vi "RT Driver VI.vi"(7 "Operation":T1, 11 "Device Reference in":T2 format="%.0x") -> (0 "Error Code":i32)   [LabVIEW 2020, in "AIM ARINC 429 Engine.lvlib" / "Custom Device.lvlib"]
uses:
  Custom Device.lvlib
  <vilib>/NI/NIVS Inline Async API/_VS Inline Async API/VS Inline Async API/VS Inline Async API.lvclass
  <vilib>/NI VeriStand/Custom Device API/Custom Device API.lvlib
  <vilib>/NI VeriStand/Custom Device Tools/Custom Device Utility Library/Custom Device Utility Library.lvlib
  <vilib>/NI VeriStand/Custom Device API/Data Reference.ctl
  <vilib>/NI VeriStand/Custom Device API/Block Data Reference.ctl
  Inline Execution Unit Runtime Information.ctl
  RTStateVariables.ctl
  Asynchronous Execution Unit Runtime Information.ctl
  Interfaces/Execution Unit/Execution Unit.lvclass
  Scripting/AIM/Constants.vi
  Scripting/AIM/AIM ARINC 429 Scripting.lvlib
  Inline Execution Unit Compiled Information.ctl
  Asynchronous Execution Unit Compiled Information.ctl
  Compiled.Settings.ctl
  <vilib>/NI VeriStand/Custom Device API/Get Item Property (Variant).vi
  Interfaces/Shared Resources/Shared Resources.lvclass
  <vilib>/NI VeriStand/Custom Device API/Custom Device Item Ref.ctl
  <vilib>/NI VeriStand/Custom Device API/Hardware Interface Driver VI Operation.ctl
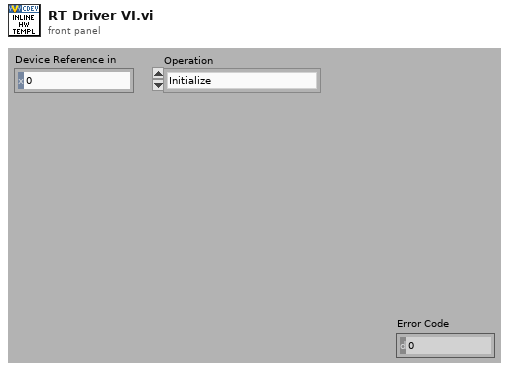
[diagram p1: front panel]
types:
  T1 = typedef "Custom Device API.lvlib/Hardware Interface Driver VI Operation.ctl" = enum16{"Initialize", "Start", "Read Data from HW", "Write Data to HW", "Close"}
  T2 = typedef "Custom Device API.lvlib/Custom Device Item Ref.ctl" = u64
  T3 = typedef "AIM ARINC 429 Engine.lvlib/Custom Device.lvlib/RTStateVariables.ctl" = cluster{"Async":refnum<class "VS Inline Async API.lvclass">, "Inline Execution Units":T4[], "Asynchronous Execution Units":T7[], "shared resources":refnum<class "Shared Resources.lvclass">}
  T4 = typedef "AIM ARINC 429 Engine.lvlib/Custom Device.lvlib/Inline Execution Unit Runtime Information.ctl" = cluster{"Execution Unit":refnum<class "Execution Unit.lvclass">, "Incoming Buffer":dbl[], "Outgoing Buffer":dbl[], "Incoming Data References":T5[], "Outgoing Data References":T6[]}
  T5 = typedef "Custom Device API.lvlib/Data Reference.ctl" = i32
  T6 = typedef "Custom Device API.lvlib/Block Data Reference.ctl" = cluster{"Data Reference":T5, "Offset":u64, "Length":u64}
  T7 = typedef "AIM ARINC 429 Engine.lvlib/Custom Device.lvlib/Asynchronous Execution Unit Runtime Information.ctl" = cluster{"Execution Unit":refnum<class "Execution Unit.lvclass">, "Incoming Channel Group Name":string, "Outgoing Channel Group Name":string, "ReadWrite Channel Group Name":string}
  T8 = typedef "AIM ARINC 429 Engine.lvlib/Custom Device.lvlib/Compiled.Settings.ctl" = cluster{"Name":string, "Inline Execution Unit Compiled Information":T9[], "Asynchronous Execution Unit Compiled Information":T10[], "flattened shared resources":string}
  T9 = typedef "AIM ARINC 429 Engine.lvlib/Custom Device.lvlib/Inline Execution Unit Compiled Information.ctl" = cluster{"Flattened Execution Unit":string, "Incoming Buffer":dbl[], "Outgoing Buffer":dbl[], "Incoming Data References":T5[], "Outgoing Data References":T6[]}
  T10 = typedef "AIM ARINC 429 Engine.lvlib/Custom Device.lvlib/Asynchronous Execution Unit Compiled Information.ctl" = cluster{"Flattened Execution Unit":string, "Incoming Channel Group Name":string, "Outgoing Channel Group Name":string, "ReadWrite Channel Group Name":string}
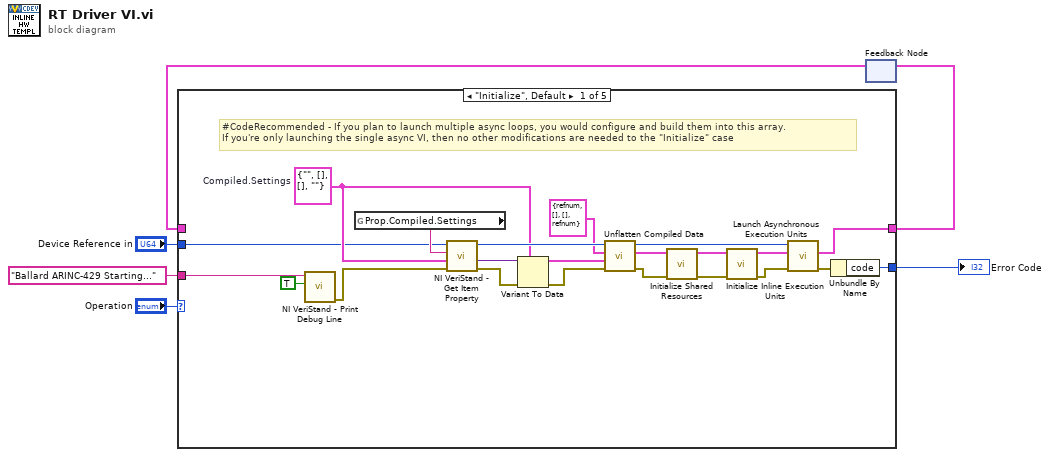
[diagram p0: block diagram]
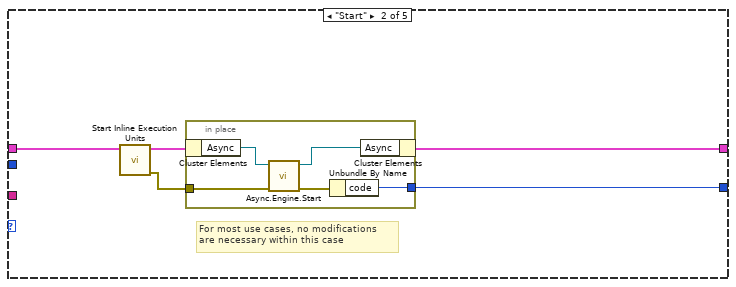
[diagram p2: hidden frame]
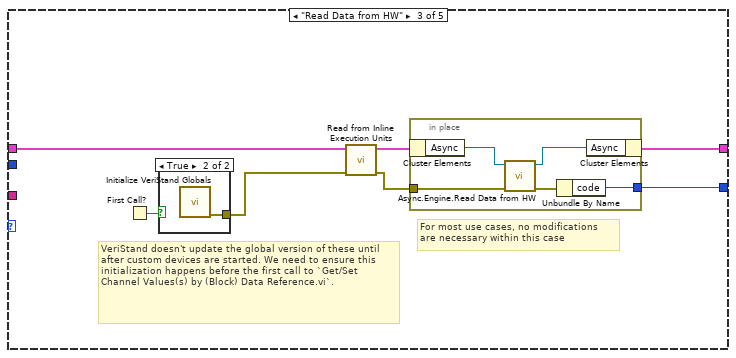
[diagram p3: hidden frame]
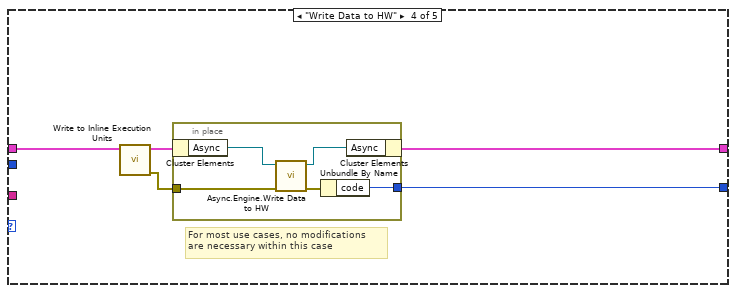
[diagram p5: hidden frame]
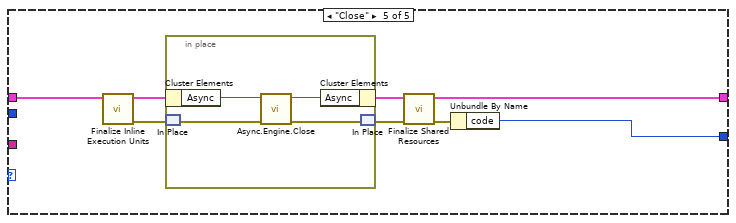
[diagram p6: hidden frame]
diagram:
  n1 = feedback #1() -> (w4:T3)  [unwired: 1 out]
  n2 = case shown="\"Initialize\", Default" "Operation" {
    tunnel: [w27 w32 w44 w55 w63] -> w5
    tunnel: w4 -> [_ w33 w43 w54 w69]
    tunnel: "Device Reference in" -> [w15 _ _ _ _]
    tunnel: [w28 w31 w45 w56 w67] -> w2
    tunnel: "Ballard ARINC-429 Starting..." ("Message") -> [w26 _ _ _ _]
    frame "Initialize", Default {
      w17 = T8 {"Name"="", "Inline Execution Unit Compiled Information"=[], "Asynchronous Execution Unit Compiled Information"=[], "flattened shared resources"=""}  # Compiled.Settings
      # "#CodeRecommended - If you plan to launch multiple async loops, you would configure and build them into this array. \nIf you're only launching the single async VI, then no other modifications are needed to the \"Initialize\" case"
      n3 = call <vilib>:"NI VeriStand - Print Debug Line.vi"("Add to log file? (F)"=TRUE, "Message"=w26) -> ("error out"=w12:errorcluster)  [unwired: 9 in]
      n4 = global read "Constants.vi" "Prop.Compiled.Settings"() -> (w16:string)
      n5 = call-poly <vilib>:"NI VeriStand - Get Item Property.vi"("error in (no error)"=w12, "Default Value"=w17, "Property Name"=w16, "Item Ref in"=w15) -> ("error out"=w21:errorcluster, "Value"=w23:variant, "Item Ref out"=w22:T2)  [unwired: 4 in, 1 out]
      n6 = Variant To Data(error in=w21, type=w17, Variant=w23) -> (data=w18:T8, error out=w10:errorcluster)
      n7 = call "Unflatten Compiled Data.vi"("error in"=w10, "Compiled.Settings"=w18, "RTStateVariables in"=T3 {"Async"=refnum, "Inline Execution Units"=[], "Asynchronous Execution Units"=[], "shared resources"=refnum} ("RTStateVariables"), "Item Ref in"=w22) -> ("error out"=w11:errorcluster, "RTStateVariables out"=w14:T3, "Item Ref out"=w24:T2)  [unwired: 5 in]
      n8 = call "Initialize Shared Resources.vi"("error in"=w11, "RTStateVariables in"=w14) -> ("error out"=w9:errorcluster, "RTStateVariables out"=w13:T3)  [unwired: 6 in]
      n9 = call "Initialize Inline Execution Units.vi"("error in"=w9, "RTStateVariables in"=w13) -> ("error out"=w8:errorcluster, "RTStateVariables out"=w25:T3)  [unwired: 8 in]
      n10 = call "Launch Asynchronous Execution Units.vi"("error in"=w8, "RTStateVariables in"=w25, "Device Ref in"=w24) -> ("error out"=w7:errorcluster, "RTStateVariables out"=w27:T3)  [unwired: 6 in, 1 out]
      n11 = Unbundle By Name(w7) -> ("code"=w28:i32)
    }
    frame "Start" {
      # "For most use cases, no modifications \nare necessary within this case"
      n12 = call "Start Inline Execution Units.vi"("RTStateVariables in"=w33) -> ("error out"=w29:errorcluster, "RTStateVariables out"=w30:T3)  [unwired: 9 in]
      n13 = in-place {
        in-place-border: [w35] -> w31
        in-place-border: w29 -> [w34]
        n14 = in-place-cluster #2(w30) -> ("Async"=w38:refnum<class "VS Inline Async API.lvclass">)
        n15 = call <vilib>:"Async.Engine.Start.vi"("error in (no error)"=w34, "VS Inline Async API in"=w38) -> ("error out"=w36:errorcluster, "VS Inline Async API out"=w37:refnum<class "VS Inline Async API.lvclass">)  [unwired: 8 in]
        n16 = Unbundle By Name(w36) -> ("code"=w35:i32)
        n17 = in-place-cluster #2("Async"=w37) -> (w32:T3)
      }
    }
    frame "Read Data from HW" {
      # "VeriStand doesn't update the global version of these until after custom devices are started. We need to ensure this initialization happens before the first call to `Get/Set Channel Values(s) by (Block) Data Reference.vi`."
      # "For most use cases, no modifications \nare necessary within this case"
      n18 = First Call?() -> (First Call?: T/F=w40:bool)
      n19 = case shown="True" w40 {
        tunnel: [_ w46] -> w39
        frame False {
        }
        frame True {
          n20 = call "Initialize VeriStand Globals.vi"() -> ("error out"=w46:errorcluster)  [unwired: 11 in]
        }
      }
      n21 = call "Read from Inline Execution Units.vi"("error in (no error)"=w39, "RTStateVariables in"=w43) -> ("error out"=w41:errorcluster, "RTStateVariables out"=w42:T3)  [unwired: 8 in]
      n22 = in-place {
        in-place-border: [w49] -> w45
        in-place-border: w41 -> [w47]
        n23 = in-place-cluster #3(w42) -> ("Async"=w51:refnum<class "VS Inline Async API.lvclass">)
        n24 = call <vilib>:"Async.Engine.Read Data from HW.vi"("error in"=w47, "Async in"=w51) -> ("error out"=w48:errorcluster, "Async out"=w50:refnum<class "VS Inline Async API.lvclass">)  [unwired: 8 in]
        n25 = Unbundle By Name(w48) -> ("code"=w49:i32)
        n26 = in-place-cluster #3("Async"=w50) -> (w44:T3)
      }
    }
    frame "Write Data to HW" {
      # "For most use cases, no modifications \nare necessary within this case"
      n27 = call "Write to Inline Execution Units.vi"("RTStateVariables in"=w54) -> ("error out"=w52:errorcluster, "RTStateVariables out"=w53:T3)  [unwired: 9 in]
      n28 = in-place {
        in-place-border: [w61] -> w56
        in-place-border: w52 -> [w57]
        n29 = in-place-cluster #4(w53) -> ("Async"=w59:refnum<class "VS Inline Async API.lvclass">)
        n30 = call <vilib>:"Async.Engine.Write Data to HW.vi"("error in (no error)"=w57, "VS Inline Async API in"=w59) -> ("error out"=w60:errorcluster, "VS Inline Async API out"=w58:refnum<class "VS Inline Async API.lvclass">)  [unwired: 8 in]
        n31 = Unbundle By Name(w60) -> ("code"=w61:i32)
        n32 = in-place-cluster #4("Async"=w58) -> (w55:T3)
      }
    }
    frame "Close" {
      n33 = call "Finalize Inline Execution Units.vi"("RTStateVariables in"=w69) -> ("error out"=w66:errorcluster, "RTStateVariables out"=w68:T3)  [unwired: 9 in]
      n34 = in-place {
        n35 = in-place-cluster #5(w68) -> ("Async"=w73:refnum<class "VS Inline Async API.lvclass">)
        n36 = in-place-match #6(w66) -> (w71:errorcluster)
        n37 = call <vilib>:"Async.Engine.Close.vi"("error in (no error)"=w71, "Async in"=w73) -> ("error out"=w70:errorcluster, "Async out"=w72:refnum<class "VS Inline Async API.lvclass">)  [unwired: 8 in]
        n38 = in-place-cluster #5("Async"=w72) -> (w64:T3)
        n39 = in-place-match #6(w70) -> (w65:errorcluster)
      }
      n40 = call "Finalize Shared Resources.vi"("error in"=w65, "RTStateVariables in"=w64) -> ("error out"=w62:errorcluster, "RTStateVariables out"=w63:T3)  [unwired: 8 in]
      n41 = Unbundle By Name(w62) -> ("code"=w67:i32)
    }
  }
  "Error Code" <- w2
  n42 = feedback-in #1(w5) -> ()
